vi "战舰弹窗.vi"() -> ()   [LabVIEW 2018]
panel:
  in  "关卡":dbl
  out "失败界面":picture
  out "胜利界面":picture
  out "敌机是否入侵":bool
  out "得分":dbl
  out "战舰爆炸":picture
  out "血量":dbl
  out "战舰血量":T1 scale=0.0..100.0
  out "敌机爆炸":picture
  in  "敌机数量":dbl
  in  "敌机速度":dbl
  out "敌机":picture
  out "按键":dbl
  out "战舰":T2
  out "激光武器1":T3
  out "激光武器 2":T3
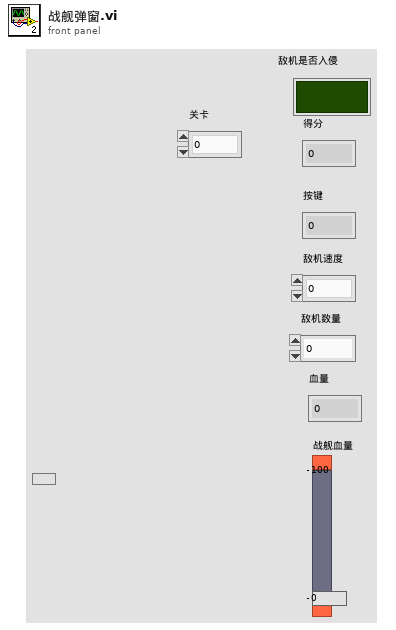
[diagram p1: front panel]
types:
  T1 = typedef "战列巡洋舰_血条.ctl" = dbl
  T2 = typedef "战列巡洋舰.ctl" = picture
  T3 = typedef "战列巡洋舰_激光武器.ctl" = picture
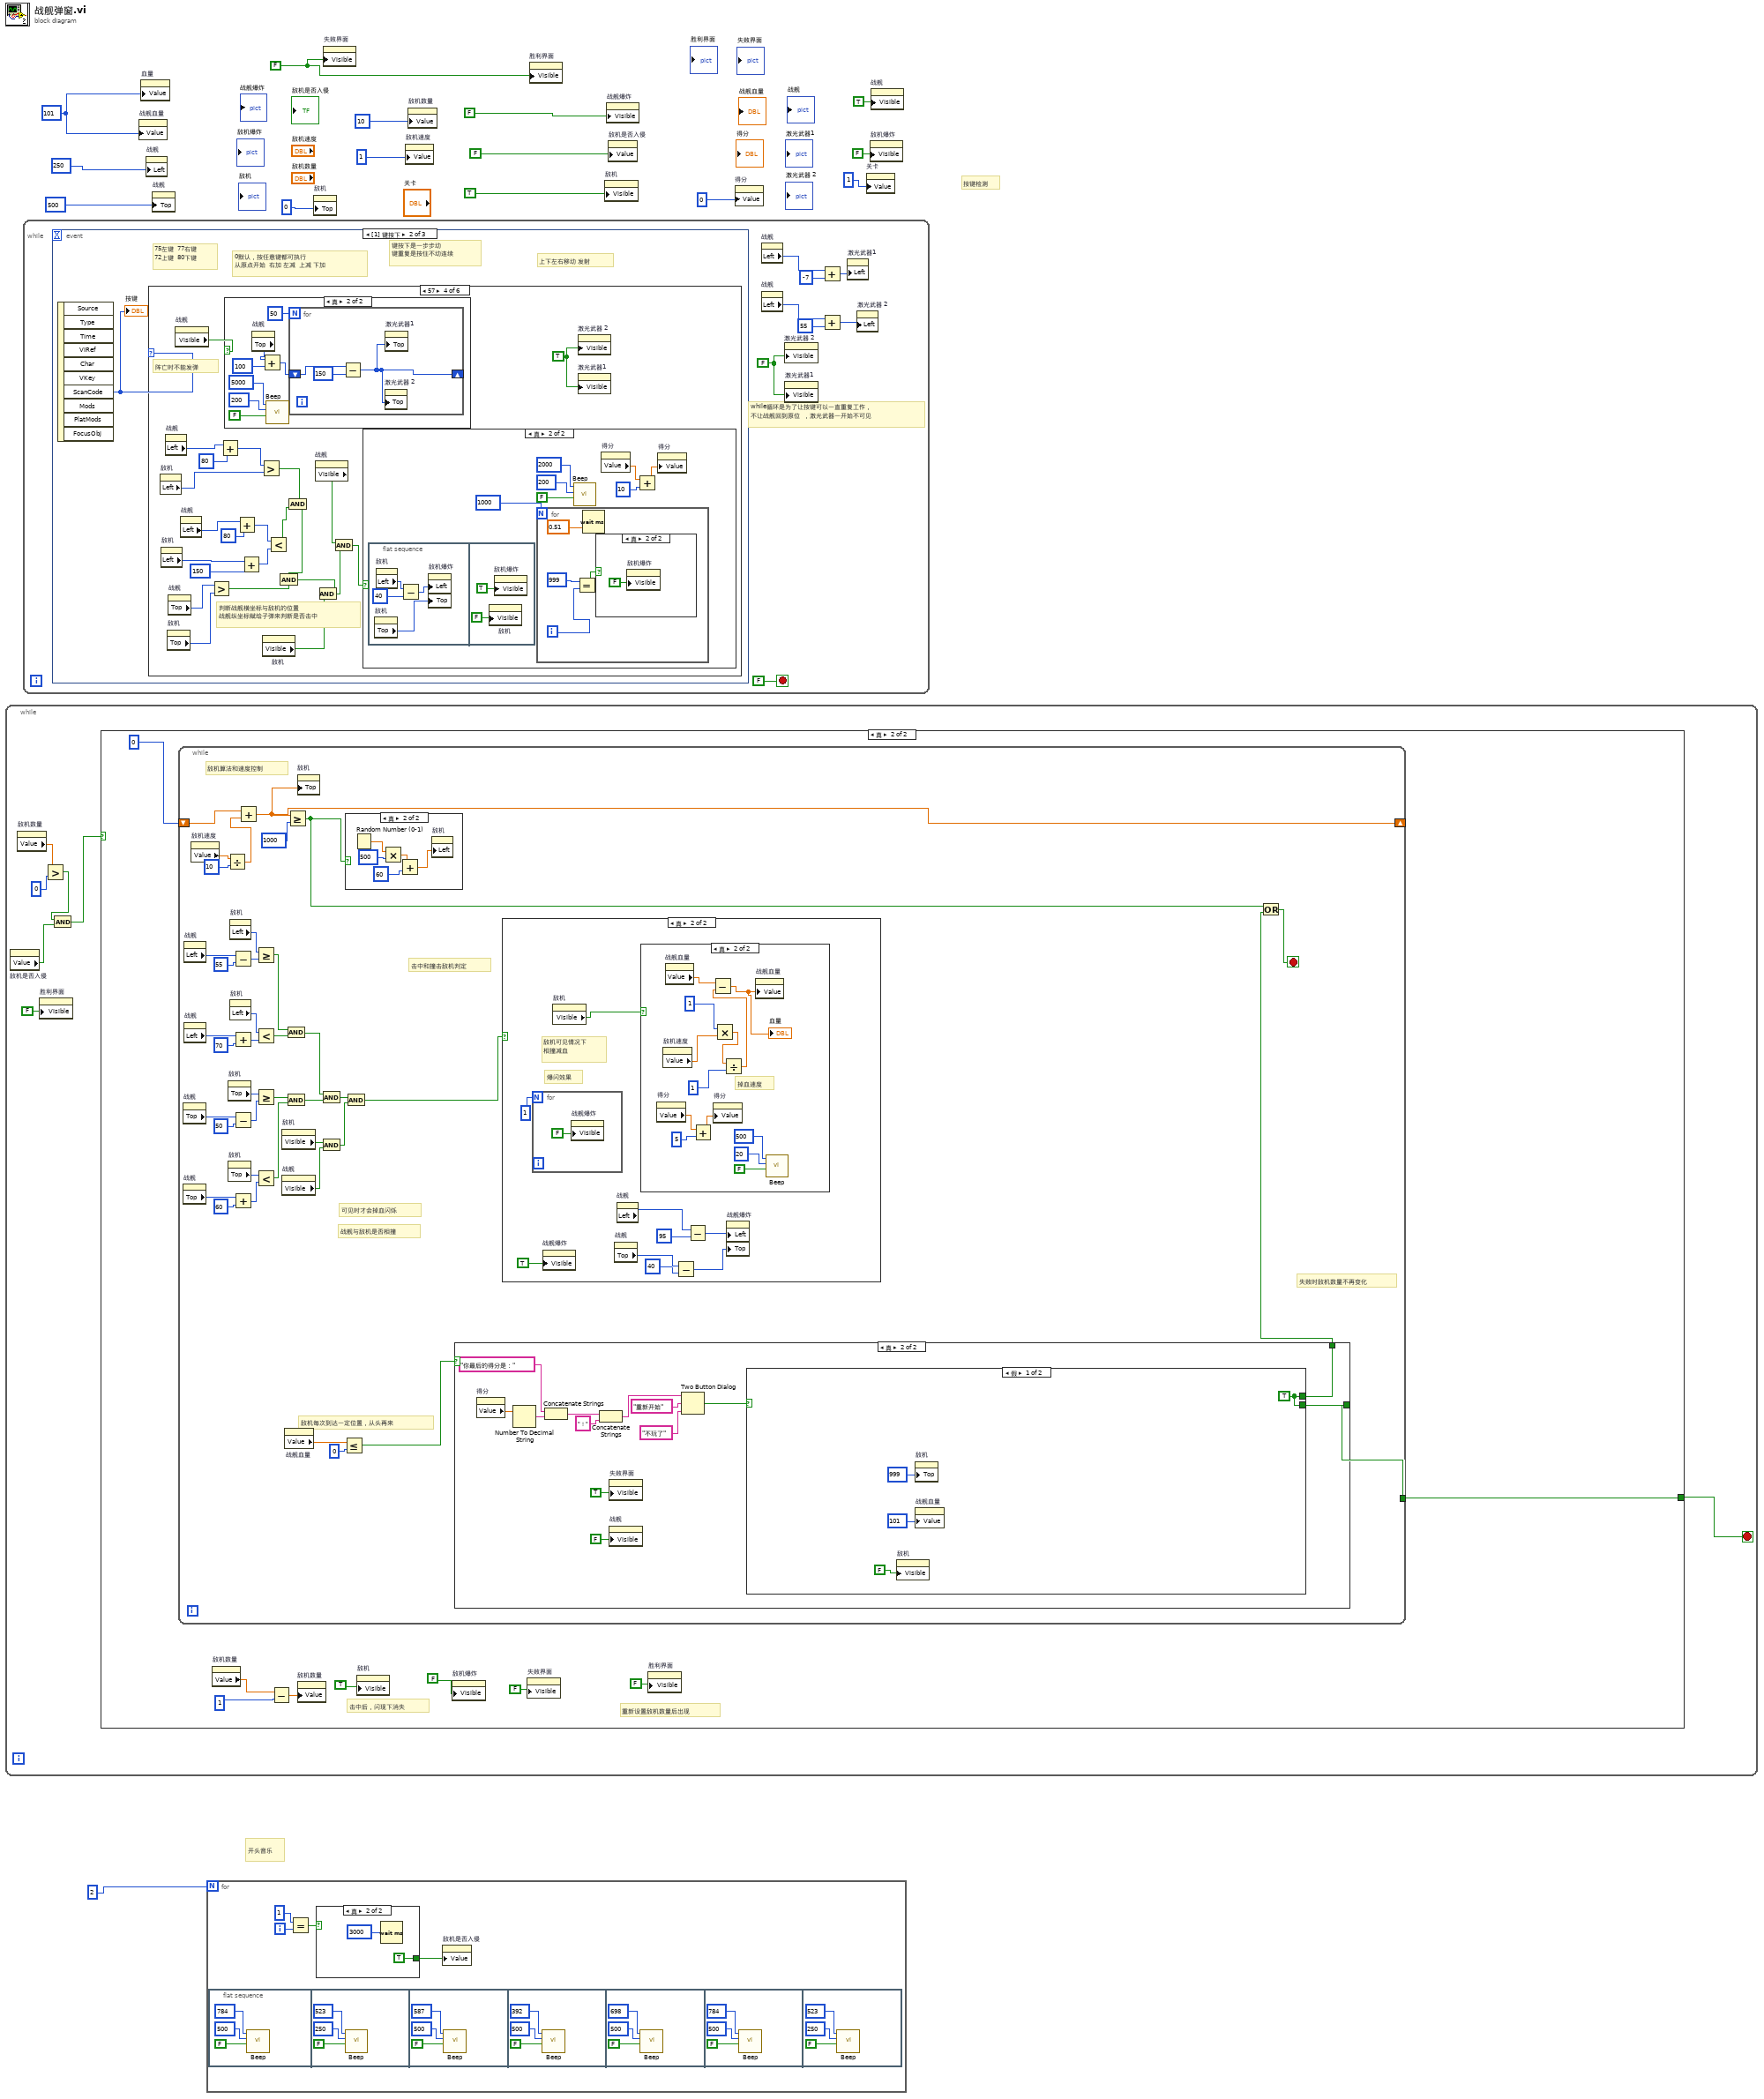
[diagram p0: block diagram]
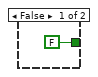
[diagram p2: hidden frame]
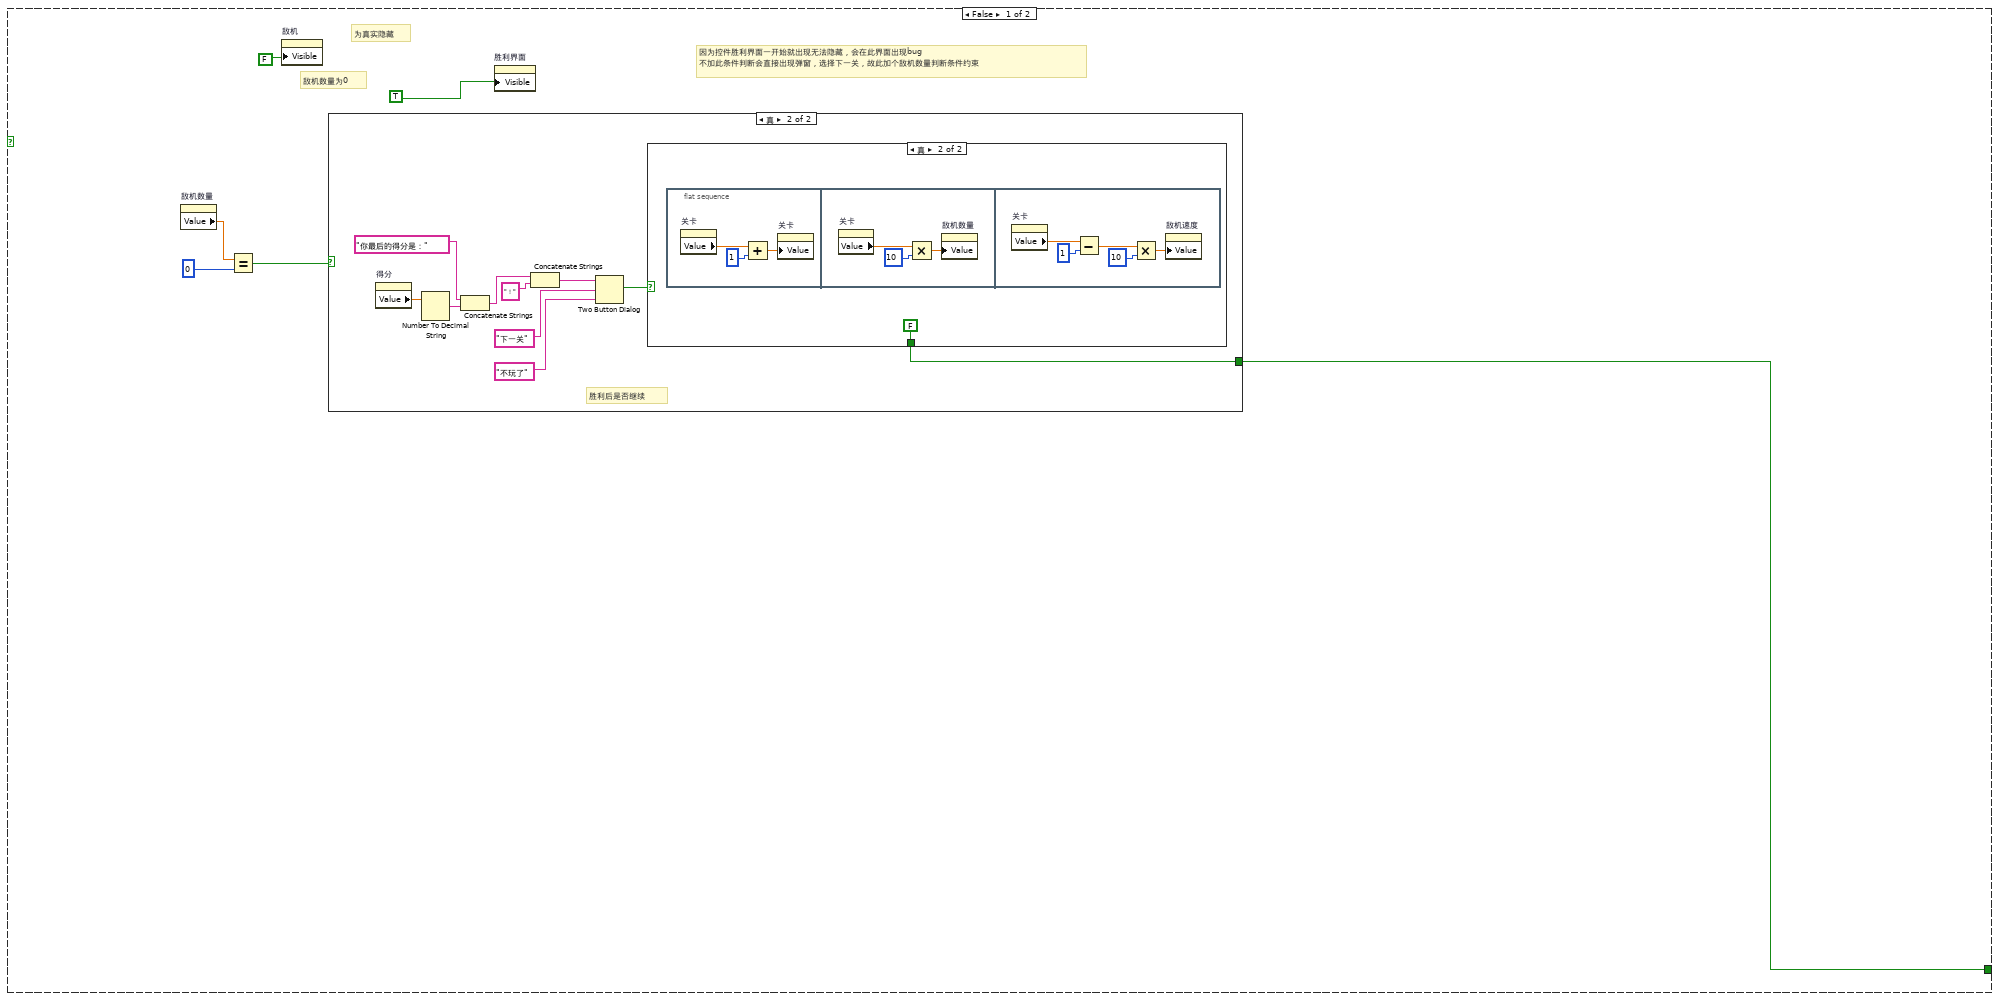
[diagram p3: hidden frame]
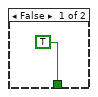
[diagram p5: hidden frame]
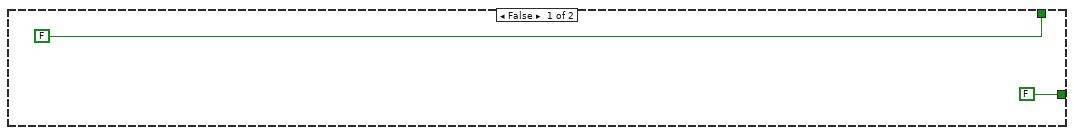
[diagram p6: hidden frame]
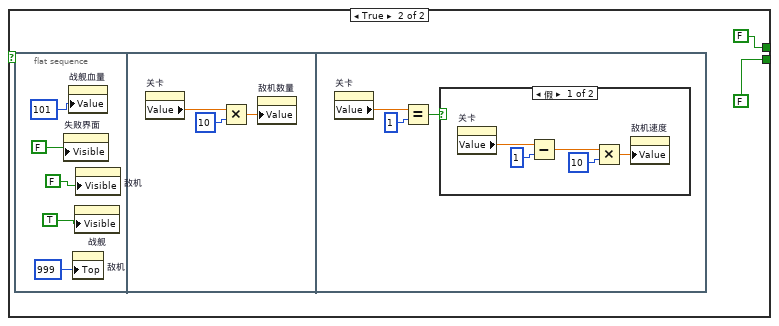
[diagram p7: hidden frame]
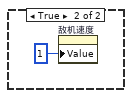
[diagram p8: hidden frame]
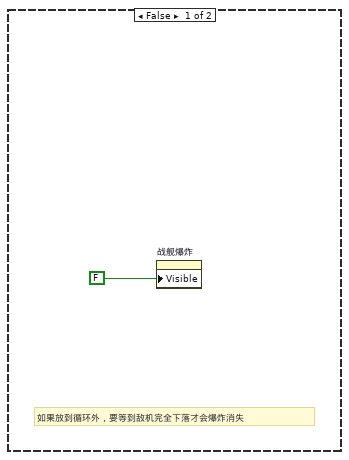
[diagram p9: hidden frame]
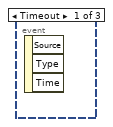
[diagram p12: hidden frame]
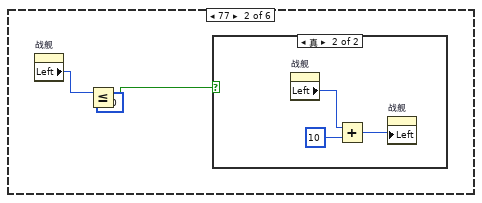
[diagram p14: hidden frame]
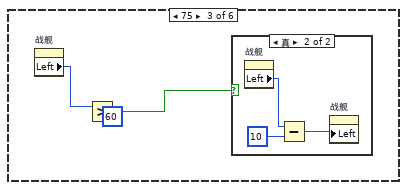
[diagram p16: hidden frame]
diagram:
  w1 = FALSE ("可见")
  w9 = 101
  # "开头音乐"
  # "按键检测"
  n1 = while {
    stop <- w17 stop-if-true
    n2 = property on="敌机是否入侵" class="Bool (严格)"() -> ("Value"=w20:bool)  [unwired: 2 in, 2 out]
    n3 = property on="敌机数量" class="DigNum (严格)"() -> ("Value"=w22:dbl)  [unwired: 2 in, 2 out]
    n4 = property on="胜利界面" class="Pict"("Visible"=FALSE ("可见")) -> ()  [unwired: 2 in, 2 out]
    n5 = Greater?(x=w22, y=0) -> (0:w19:bool)
    n6 = And(x=w19, y=w20) -> (x .and. y?=w18:bool)
    n7 = case shown="真" w18 {
      tunnel: [w26 w53] -> w17
      frame False {
        # "因为控件胜利界面一开始就出现无法隐藏，会在此界面出现bug\n不加此条件判断会直接出现弹窗，选择下一关，故此加个敌机数量判断条件约束"
        # "敌机数量为0"
        # "为真实隐藏"
        n8 = property on="敌机数量" class="DigNum (严格)"() -> ("Value"=w25:dbl)  [unwired: 2 in, 2 out]
        n9 = Equal?(x=w25, y=0) -> (x = y?=w23:bool)
        n10 = property on="敌机" class="Pict"("Visible"=FALSE ("可见")) -> ()  [unwired: 2 in, 2 out]
        n11 = case shown="真" w23 {
          tunnel: [_ w29] -> w26
          frame False {
          }
          frame True {
            # "胜利后是否继续"
            n12 = property on="得分" class="DigNum (严格)"() -> ("Value"=w37:dbl)  [unwired: 2 in, 2 out]
            n13 = Number To Decimal String(number=w37) -> (decimal integer string=w35:string)  [unwired: 1 in]
            n14 = Concatenate Strings("你最后的得分是：", w35) -> (w34:string)
            n15 = Concatenate Strings(w34, "！") -> (w32:string)
            n16 = Two Button Dialog(message=w32, 1:"不玩了" ("F按钮名称（“取消”）"), 2:"下一关" ("T按钮名称（“确定”）")) -> (T button?=w38:bool)
            n17 = case shown="真" w38 {
              tunnel: [TRUE FALSE] -> w29
              frame False {
              }
              frame True {
                n18 = flat-sequence {
                  frame #0 {
                    n19 = property on="关卡" class="DigNum (严格)"() -> ("Value"=w43:dbl)  [unwired: 2 in, 2 out]
                    n20 = Add(x=w43, y=1) -> (x+y=w41:dbl)
                    n21 = property on="关卡" class="DigNum (严格)"("Value"=w41) -> ()  [unwired: 2 in, 2 out]
                  }
                  frame #1 {
                    n22 = property on="关卡" class="DigNum (严格)"() -> ("Value"=w45:dbl)  [unwired: 2 in, 2 out]
                    n23 = Multiply(x=w45, y=10) -> (x*y=w46:dbl)
                    n24 = property on="敌机数量" class="DigNum (严格)"("Value"=w46) -> ()  [unwired: 2 in, 2 out]
                  }
                  frame #2 {
                    n25 = property on="关卡" class="DigNum (严格)"() -> ("Value"=w50:dbl)  [unwired: 2 in, 2 out]
                    n26 = Subtract(x=w50, y=1) -> (x-y=w48:dbl)
                    n27 = Multiply(x=w48, y=10) -> (x*y=w47:dbl)
                    n28 = property on="敌机速度" class="DigNum (严格)"("Value"=w47) -> ()  [unwired: 2 in, 2 out]
                  }
                }
              }
            }
          }
        }
        n29 = property on="胜利界面" class="Pict"("Visible"=TRUE ("可见")) -> ()  [unwired: 2 in, 2 out]
      }
      frame True {
        # "重新设置敌机数量后出现"
        # "击中后，闪现下消失"
        # "敌机每次到达一定位置，从头再来"
        n30 = while {
          shift-right: [w98] -> _
          shift-left: 0 -> [w100]
          tunnel: [w64] -> w53
          stop <- w62 stop-if-true
          # "失败时敌机数量不再变化"
          # "击中和撞击敌机判定"
          # "可见时才会掉血闪烁"
          # "战舰与敌机是否相撞"
          # "敌机算法和速度控制"
          n31 = property on="战舰" class="Pict (严格)"() -> ("Top"=w83:i32)  [unwired: 2 in, 2 out]
          n32 = property on="战舰" class="Pict (严格)"() -> ("Top"=w77:i32)  [unwired: 2 in, 2 out]
          n33 = property on="战舰" class="Pict (严格)"() -> ("Left"=w93:i32)  [unwired: 2 in, 2 out]
          n34 = property on="战舰" class="Pict (严格)"() -> ("Left"=w87:i32)  [unwired: 2 in, 2 out]
          n35 = property on="敌机速度" class="DigNum (严格)"() -> ("Value"=w97:dbl)  [unwired: 2 in, 2 out]
          n36 = Divide(x=w97, y=10) -> (x/y=w96:dbl)
          n37 = property on="敌机" class="Pict"() -> ("Top"=w84:i32)  [unwired: 2 in, 2 out]
          n38 = property on="敌机" class="Pict"() -> ("Top"=w76:i32)  [unwired: 2 in, 2 out]
          n39 = property on="敌机" class="Pict"() -> ("Left"=w94:i32)  [unwired: 2 in, 2 out]
          n40 = property on="敌机" class="Pict"() -> ("Left"=w89:i32)  [unwired: 2 in, 2 out]
          n41 = Subtract(x=w93, y=55) -> (x-y=w92:i32)
          n42 = Add(x=w87, y=70) -> (x+y=w86:i32)
          n43 = Subtract(x=w83, y=50) -> (x-y=w81:i32)
          n44 = Add(x=w77, y=60) -> (x+y=w79:i32)
          n45 = Add(x=w100, y=w96) -> (x+y=w98:dbl)
          n46 = Greater Or Equal?(x=w94, y=w92) -> (x >= y?=w90:bool)
          n47 = Less?(x=w89, y=w86) -> (x < y?=w85:bool)
          n48 = Greater Or Equal?(x=w84, y=w81) -> (x >= y?=w75:bool)
          n49 = Less?(x=w76, y=w79) -> (x < y?=w74:bool)
          n50 = property on="敌机" class="Pict"() -> ("Visible"=w67:bool)  [unwired: 2 in, 2 out]
          n51 = property on="战舰" class="Pict (严格)"() -> ("Visible"=w66:bool)  [unwired: 2 in, 2 out]
          n52 = And(x=w90, y=w85) -> (x .and. y?=w80:bool)
          n53 = And(x=w75, y=w74) -> (x .and. y?=w73:bool)
          n54 = property on="战舰血量" class="Slide (严格)"() -> ("Value"=w69:T1)  [unwired: 2 in, 2 out]
          n55 = Greater Or Equal?(x=w98, y=1000) -> (x >= y?=w63:bool)
          n56 = property on="敌机" class="Pict"("Top"=w98) -> ()  [unwired: 2 in, 2 out]
          n57 = And(x=w80, y=w73) -> (x .and. y?=w72:bool)
          n58 = And(x=w67, y=w66) -> (x .and. y?=w65:bool)
          n59 = Less Or Equal?(x=w69, y=0) -> (x <= y?=w70:bool)
          n60 = case shown="真" w63 {
            frame False {
            }
            frame True {
              n61 = Random Number (0-1)() -> (number: 0 to 1=w167:dbl)
              n62 = Multiply(x=w167, y=500) -> (x*y=w165:dbl)
              n63 = Add(x=w165, y=60) -> (x+y=w164:dbl)
              n64 = property on="敌机" class="Pict"("Left"=w164) -> ()  [unwired: 2 in, 2 out]
            }
          }
          n65 = And(x=w72, y=w65) -> (x .and. y?=w71:bool)
          n66 = case shown="真" w70 {
            tunnel: [FALSE w104] -> w64
            tunnel: [FALSE w103] -> w61
            frame False {
            }
            frame True {
              n67 = property on="得分" class="DigNum (严格)"() -> ("Value"=w115:dbl)  [unwired: 2 in, 2 out]
              n68 = Number To Decimal String(number=w115) -> (decimal integer string=w114:string)  [unwired: 1 in]
              n69 = Concatenate Strings("你最后的得分是：", w114) -> (w113:string)
              n70 = Concatenate Strings(w113, "！") -> (w112:string)
              n71 = property on="失败界面" class="Pict"("Visible"=TRUE ("可见")) -> ()  [unwired: 2 in, 2 out]
              n72 = property on="战舰" class="Pict (严格)"("Visible"=FALSE ("可见")) -> ()  [unwired: 2 in, 2 out]
              n73 = Two Button Dialog(message=w112, 1:"不玩了" ("F按钮名称（“取消”）"), 2:"重新开始" ("T按钮名称（“确定”）")) -> (T button?=w107:bool)
              n74 = case shown="假" w107 {
                tunnel: [w117 FALSE] -> w104
                tunnel: [w117 FALSE] -> w103
                frame False {
                  w117 = TRUE
                  n75 = property on="敌机" class="Pict"("Visible"=FALSE ("可见")) -> ()  [unwired: 2 in, 2 out]
                  n76 = property on="敌机" class="Pict"("Top"=999 ("位置:置顶")) -> ()  [unwired: 2 in, 2 out]
                  n77 = property on="战舰血量" class="Slide (严格)"("Value"=101) -> ()  [unwired: 2 in, 2 out]
                }
                frame True {
                  n78 = flat-sequence {
                    frame #0 {
                      n79 = property on="失败界面" class="Pict"("Visible"=FALSE ("可见")) -> ()  [unwired: 2 in, 2 out]
                      n80 = property on="战舰血量" class="Slide (严格)"("Value"=101) -> ()  [unwired: 2 in, 2 out]
                      n81 = property on="敌机" class="Pict"("Top"=999 ("位置:置顶")) -> ()  [unwired: 2 in, 2 out]
                      n82 = property on="战舰" class="Pict (严格)"("Visible"=TRUE ("可见")) -> ()  [unwired: 2 in, 2 out]
                      n83 = property on="敌机" class="Pict"("Visible"=FALSE ("可见")) -> ()  [unwired: 2 in, 2 out]
                    }
                    frame #1 {
                      n84 = property on="关卡" class="DigNum (严格)"() -> ("Value"=w127:dbl)  [unwired: 2 in, 2 out]
                      n85 = Multiply(x=w127, y=10) -> (x*y=w129:dbl)
                      n86 = property on="敌机数量" class="DigNum (严格)"("Value"=w129) -> ()  [unwired: 2 in, 2 out]
                    }
                    frame #2 {
                      n87 = property on="关卡" class="DigNum (严格)"() -> ("Value"=w132:dbl)  [unwired: 2 in, 2 out]
                      n88 = Equal?(x=w132, y=1) -> (x = y?=w130:bool)
                      n89 = case shown="假" w130 {
                        frame False {
                          n90 = property on="关卡" class="DigNum (严格)"() -> ("Value"=w136:dbl)  [unwired: 2 in, 2 out]
                          n91 = Subtract(x=w136, y=1) -> (x-y=w133:dbl)
                          n92 = Multiply(x=w133, y=10) -> (x*y=w137:dbl)
                          n93 = property on="敌机速度" class="DigNum (严格)"("Value"=w137) -> ()  [unwired: 2 in, 2 out]
                        }
                        frame True {
                          n94 = property on="敌机速度" class="DigNum (严格)"("Value"=1) -> ()  [unwired: 2 in, 2 out]
                        }
                      }
                    }
                  }
                }
              }
            }
          }
          n95 = case shown="真" w71 {
            frame False {
              # "如果放到循环外，要等到敌机完全下落才会爆炸消失"
              n96 = property on="战舰爆炸" class="Pict"("Visible"=FALSE ("可见")) -> ()  [unwired: 2 in, 2 out]
            }
            frame True {
              # "爆闪效果"
              # "敌机可见情况下\n相撞减血"
              n97 = for {
                N: 1 -> [_]
                n98 = property on="战舰爆炸" class="Pict"("Visible"=FALSE ("可见")) -> ()  [unwired: 2 in, 2 out]
              }
              n99 = property on="战舰爆炸" class="Pict"("Visible"=TRUE ("可见")) -> ()  [unwired: 2 in, 2 out]
              n100 = property on="敌机" class="Pict"() -> ("Visible"=w148:bool)  [unwired: 2 in, 2 out]
              n101 = property on="战舰" class="Pict (严格)"() -> ("Top"=w143:i32)  [unwired: 2 in, 2 out]
              n102 = property on="战舰" class="Pict (严格)"() -> ("Left"=w146:i32)  [unwired: 2 in, 2 out]
              n103 = case shown="真" w148 {
                frame False {
                }
                frame True {
                  # "掉血速度"
                  n104 = property on="得分" class="DigNum (严格)"() -> ("Value"=w155:dbl)  [unwired: 2 in, 2 out]
                  n105 = property on="敌机速度" class="DigNum (严格)"() -> ("Value"=w161:dbl)  [unwired: 2 in, 2 out]
                  n106 = property on="战舰血量" class="Slide (严格)"() -> ("Value"=w162:T1)  [unwired: 2 in, 2 out]
                  n107 = Add(x=w155, y=5) -> (x+y=w154:dbl)
                  n108 = Multiply(x=1, y=w161) -> (x*y=w160:dbl)
                  n109 = property on="得分" class="DigNum (严格)"("Value"=w154) -> ()  [unwired: 2 in, 2 out]
                  n110 = Divide(x=w160, y=1) -> (x/y=w157:dbl)
                  n111 = Subtract(x=w162, y=w157) -> (x-y=w156:T1)
                  "血量" <- w156
                  n112 = property on="战舰血量" class="Slide (严格)"("Value"=w156) -> ()  [unwired: 2 in, 2 out]
                  n113 = call <vilib>:"Beep.vi"("use system alert? (T)"=FALSE, "duration (msec)"=u32 20, "frequency (Hz)"=u32 500) -> ()  [unwired: 9 in]
                }
              }
              n114 = Subtract(x=w143, y=40) -> (x-y=w141:i32)
              n115 = Subtract(x=w146, y=95) -> (x-y=w144:i32)
              n116 = property on="战舰爆炸" class="Pict"("Left"=w144, "Top"=w141) -> ()  [unwired: 2 in, 2 out]
            }
          }
          n117 = Or(x=w63, y=w61) -> (x .or. y?=w62:bool)
        }
        n118 = property on="敌机数量" class="DigNum (严格)"() -> ("Value"=w58:dbl)  [unwired: 2 in, 2 out]
        n119 = Subtract(x=w58, y=1) -> (x-y=w59:dbl)
        n120 = property on="敌机数量" class="DigNum (严格)"("Value"=w59) -> ()  [unwired: 2 in, 2 out]
        n121 = property on="敌机" class="Pict"("Visible"=TRUE ("可见")) -> ()  [unwired: 2 in, 2 out]
        n122 = property on="敌机爆炸" class="Pict"("Visible"=FALSE ("可见")) -> ()  [unwired: 2 in, 2 out]
        n123 = property on="失败界面" class="Pict"("Visible"=FALSE ("可见")) -> ()  [unwired: 2 in, 2 out]
        n124 = property on="胜利界面" class="Pict"("Visible"=FALSE ("可见")) -> ()  [unwired: 2 in, 2 out]
      }
    }
  }
  n125 = while {
    stop <- FALSE stop-if-true
    w168 = FALSE
    # "while循环是为了让按键可以一直重复工作，\n不让战舰回到原位  ，激光武器一开始不可见"
    n126 = event shown="[1] 键按下" {
      selector: _ -> [_ _ _]
      dyn-events: _ -> [_ _ _]
      timeout: _ -> [_ _ _]
      event Timeout {
        n127 = event-data() -> ()  [unwired: 1 in, 3 out]
      }
      event Key Down {
        # "上下左右移动 发射"
        # "键按下是一步步动\n键重复是按住不动连续"
        # "75左键  77右键\n72上键  80下键"
        # "0默认，按任意键都可执行\n从原点开始  右加 左减  上减 下加"
        n128 = event-data() -> ("ScanCode"=w176:i16)  [unwired: 1 in, 9 out]
        "按键" <- w176
        n129 = case shown="57" w176 {
          frame 0, Default {
          }
          frame 77 {
            n130 = property on="战舰" class="Pict (严格)"() -> ("Left"=w179:i32)  [unwired: 2 in, 2 out]
            n131 = Less Or Equal?(x=w179, y=500) -> (x <= y?=w177:bool)
            n132 = case shown="真" w177 {
              frame False {
              }
              frame True {
                n133 = property on="战舰" class="Pict (严格)"() -> ("Left"=w181:i32)  [unwired: 2 in, 2 out]
                n134 = Add(x=w181, y=10) -> (x+y=w182:i32)
                n135 = property on="战舰" class="Pict (严格)"("Left"=w182) -> ()  [unwired: 2 in, 2 out]
              }
            }
          }
          frame 75 {
            n136 = property on="战舰" class="Pict (严格)"() -> ("Left"=w185:i32)  [unwired: 2 in, 2 out]
            n137 = Greater?(x=w185, y=60) -> (0:w183:bool)
            n138 = case shown="真" w183 {
              frame False {
              }
              frame True {
                n139 = property on="战舰" class="Pict (严格)"() -> ("Left"=w187:i32)  [unwired: 2 in, 2 out]
                n140 = Subtract(x=w187, y=10) -> (x-y=w188:i32)
                n141 = property on="战舰" class="Pict (严格)"("Left"=w188) -> ()  [unwired: 2 in, 2 out]
              }
            }
          }
          frame 57 {
            w211 = TRUE
            # "阵亡时不能发弹"
            # "判断战舰横坐标与敌机的位置\n战舰纵坐标赋给子弹来判断是否击中"
            n142 = property on="敌机" class="Pict"() -> ("Left"=w208:i32)  [unwired: 2 in, 2 out]
            n143 = property on="敌机" class="Pict"() -> ("Left"=w201:i32)  [unwired: 2 in, 2 out]
            n144 = property on="战舰" class="Pict (严格)"() -> ("Left"=w210:i32)  [unwired: 2 in, 2 out]
            n145 = property on="敌机" class="Pict"() -> ("Top"=w195:i32)  [unwired: 2 in, 2 out]
            n146 = property on="战舰" class="Pict (严格)"() -> ("Top"=w196:i32)  [unwired: 2 in, 2 out]
            n147 = property on="战舰" class="Pict (严格)"() -> ("Visible"=w189:bool)  [unwired: 2 in, 2 out]
            n148 = property on="战舰" class="Pict (严格)"() -> ("Left"=w203:i32)  [unwired: 2 in, 2 out]
            n149 = Greater?(x=w196, y=w195) -> (0:w197:bool)
            n150 = Add(x=w210, y=80) -> (x+y=w207:i32)
            n151 = case shown="真" w189 {
              frame False {
              }
              frame True {
                n152 = property on="战舰" class="Pict (严格)"() -> ("Top"=w217:i32)  [unwired: 2 in, 2 out]
                n153 = Add(x=w217, y=100) -> (x+y=w215:i32)
                n154 = call <vilib>:"Beep.vi"("use system alert? (T)"=FALSE, "duration (msec)"=u32 200, "frequency (Hz)"=u32 5000) -> ()  [unwired: 9 in]
                n155 = for {
                  N: 50 -> [_]
                  shift-right: [w219] -> _
                  shift-left: w215 -> [w221]
                  n156 = Subtract(x=w221, y=150) -> (x-y=w219:i32)
                  n157 = property on="激光武器 2" class="Pict (严格)"("Top"=w219) -> ()  [unwired: 2 in, 2 out]
                  n158 = property on="激光武器1" class="Pict (严格)"("Top"=w219) -> ()  [unwired: 2 in, 2 out]
                }
              }
            }
            n159 = Add(x=w203, y=80) -> (x+y=w205:i32)
            n160 = Add(x=w201, y=150) -> (x+y=w200:i32)
            n161 = Greater?(x=w207, y=w208) -> (0:w206:bool)
            n162 = property on="敌机" class="Pict"() -> ("Visible"=w193:bool)  [unwired: 2 in, 2 out]
            n163 = Less?(x=w205, y=w200) -> (x < y?=w202:bool)
            n164 = And(x=w206, y=w202) -> (x .and. y?=w198:bool)
            n165 = And(x=w198, y=w197) -> (x .and. y?=w194:bool)
            n166 = property on="战舰" class="Pict (严格)"() -> ("Visible"=w192:bool)  [unwired: 2 in, 2 out]
            n167 = And(x=w194, y=w193) -> (x .and. y?=w191:bool)
            n168 = And(x=w192, y=w191) -> (x .and. y?=w190:bool)
            n169 = case shown="真" w190 {
              frame False {
              }
              frame True {
                n170 = flat-sequence {
                  frame #0 {
                    n171 = property on="敌机" class="Pict"() -> ("Top"=w232:i32)  [unwired: 2 in, 2 out]
                    n172 = property on="敌机" class="Pict"() -> ("Left"=w230:i32)  [unwired: 2 in, 2 out]
                    n173 = Subtract(x=w230, y=40) -> (x-y=w229:i32)
                    n174 = property on="敌机爆炸" class="Pict"("Left"=w229, "Top"=w232) -> ()  [unwired: 2 in, 2 out]
                  }
                  frame #1 {
                    n175 = property on="敌机" class="Pict"("Visible"=FALSE ("可见")) -> ()  [unwired: 2 in, 2 out]
                    n176 = property on="敌机爆炸" class="Pict"("Visible"=TRUE ("可见")) -> ()  [unwired: 2 in, 2 out]
                  }
                }
                n177 = for {
                  N: 1000 -> [_]
                  i -> [w237]
                  n178 = Equal?(x=999, y=w237) -> (x = y?=w238:bool)
                  n179 = Wait (ms)(milliseconds to wait=0.51) -> ()  [unwired: 1 out]
                  n180 = case shown="真" w238 {
                    frame False {
                    }
                    frame True {
                      n181 = property on="敌机爆炸" class="Pict"("Visible"=FALSE ("可见")) -> ()  [unwired: 2 in, 2 out]
                    }
                  }
                }
                n182 = call <vilib>:"Beep.vi"("use system alert? (T)"=FALSE, "duration (msec)"=u32 200, "frequency (Hz)"=u32 2000) -> ()  [unwired: 9 in]
                n183 = property on="得分" class="DigNum (严格)"() -> ("Value"=w227:dbl)  [unwired: 2 in, 2 out]
                n184 = Add(x=w227, y=10) -> (x+y=w225:dbl)
                n185 = property on="得分" class="DigNum (严格)"("Value"=w225) -> ()  [unwired: 2 in, 2 out]
              }
            }
            n186 = property on="激光武器 2" class="Pict (严格)"("Visible"=w211) -> ()  [unwired: 2 in, 2 out]
            n187 = property on="激光武器1" class="Pict (严格)"("Visible"=w211) -> ()  [unwired: 2 in, 2 out]
          }
          frame 80 {
            n188 = property on="战舰" class="Pict (严格)"() -> ("Top"=w242:i32)  [unwired: 2 in, 2 out]
            n189 = Less?(x=w242, y=525) -> (x < y?=w240:bool)
            n190 = case shown="真" w240 {
              frame False {
              }
              frame True {
                n191 = property on="战舰" class="Pict (严格)"() -> ("Top"=w244:i32)  [unwired: 2 in, 2 out]
                n192 = Add(x=w244, y=10) -> (x+y=w243:i32)
                n193 = property on="战舰" class="Pict (严格)"("Top"=w243) -> ()  [unwired: 2 in, 2 out]
              }
            }
          }
          frame 72 {
            n194 = property on="战舰" class="Pict (严格)"() -> ("Top"=w248:i32)  [unwired: 2 in, 2 out]
            n195 = Greater Or Equal?(x=w248, y=25) -> (x >= y?=w247:bool)
            n196 = case shown="真" w247 {
              frame False {
              }
              frame True {
                n197 = property on="战舰" class="Pict (严格)"() -> ("Top"=w251:i32)  [unwired: 2 in, 2 out]
                n198 = Subtract(x=w251, y=10) -> (x-y=w250:i32)
                n199 = property on="战舰" class="Pict (严格)"("Top"=w250) -> ()  [unwired: 2 in, 2 out]
              }
            }
          }
        }
      }
      event Key Repeat {
        # "75左键  77右键\n72上键  80下键\n空格 57"
        # "0默认，按任意键都可执行\n从原点开始  右加 左减  上减 下加"
        n200 = event-data() -> ("ScanCode"=w252:i16)  [unwired: 1 in, 9 out]
        n201 = case shown="72" w252 {
          frame 0, Default {
          }
          frame 77 {
            n202 = property on="战舰" class="Pict (严格)"() -> ("Left"=w255:i32)  [unwired: 2 in, 2 out]
            n203 = Less Or Equal?(x=w255, y=500) -> (x <= y?=w254:bool)
            n204 = case shown="真" w254 {
              frame False {
              }
              frame True {
                n205 = property on="战舰" class="Pict (严格)"() -> ("Left"=w257:i32)  [unwired: 2 in, 2 out]
                n206 = Add(x=w257, y=10) -> (x+y=w258:i32)
                n207 = property on="战舰" class="Pict (严格)"("Left"=w258) -> ()  [unwired: 2 in, 2 out]
              }
            }
          }
          frame 75 {
            n208 = property on="战舰" class="Pict (严格)"() -> ("Left"=w261:i32)  [unwired: 2 in, 2 out]
            n209 = Greater Or Equal?(x=w261, y=25) -> (x >= y?=w260:bool)
            n210 = case shown="真" w260 {
              frame False {
              }
              frame True {
                n211 = property on="战舰" class="Pict (严格)"() -> ("Left"=w264:i32)  [unwired: 2 in, 2 out]
                n212 = Subtract(x=w264, y=10) -> (x-y=w263:i32)
                n213 = property on="战舰" class="Pict (严格)"("Left"=w263) -> ()  [unwired: 2 in, 2 out]
              }
            }
          }
          frame 80 {
            n214 = property on="战舰" class="Pict (严格)"() -> ("Top"=w267:i32)  [unwired: 2 in, 2 out]
            n215 = Less Or Equal?(x=w267, y=525) -> (x <= y?=w266:bool)
            n216 = case shown="真" w266 {
              frame False {
              }
              frame True {
                n217 = property on="战舰" class="Pict (严格)"() -> ("Top"=w269:i32)  [unwired: 2 in, 2 out]
                n218 = Add(x=w269, y=10) -> (x+y=w268:i32)
                n219 = property on="战舰" class="Pict (严格)"("Top"=w268) -> ()  [unwired: 2 in, 2 out]
              }
            }
          }
          frame 72 {
            n220 = property on="战舰" class="Pict (严格)"() -> ("Top"=w273:i32)  [unwired: 2 in, 2 out]
            n221 = Greater Or Equal?(x=w273, y=25) -> (x >= y?=w272:bool)
            n222 = case shown="真" w272 {
              frame False {
              }
              frame True {
                n223 = property on="战舰" class="Pict (严格)"() -> ("Top"=w276:i32)  [unwired: 2 in, 2 out]
                n224 = Subtract(x=w276, y=10) -> (x-y=w275:i32)
                n225 = property on="战舰" class="Pict (严格)"("Top"=w275) -> ()  [unwired: 2 in, 2 out]
              }
            }
          }
        }
      }
    }
    n226 = property on="战舰" class="Pict (严格)"() -> ("Left"=w174:i32)  [unwired: 2 in, 2 out]
    n227 = property on="战舰" class="Pict (严格)"() -> ("Left"=w170:i32)  [unwired: 2 in, 2 out]
    n228 = property on="激光武器 2" class="Pict (严格)"("Visible"=w168) -> ()  [unwired: 2 in, 2 out]
    n229 = property on="激光武器1" class="Pict (严格)"("Visible"=w168) -> ()  [unwired: 2 in, 2 out]
    n230 = Add(x=w174, y=-7) -> (x+y=w173:i32)
    n231 = Add(x=w170, y=55) -> (x+y=w169:i32)
    n232 = property on="激光武器1" class="Pict (严格)"("Left"=w173) -> ()  [unwired: 2 in, 2 out]
    n233 = property on="激光武器 2" class="Pict (严格)"("Left"=w169) -> ()  [unwired: 2 in, 2 out]
  }
  n234 = property on="战舰血量" class="Slide (严格)"("Value"=w9) -> ()  [unwired: 2 in, 2 out]
  n235 = property on="血量" class="DigNum (严格)"("Value"=w9) -> ()  [unwired: 2 in, 2 out]
  n236 = property on="战舰" class="Pict (严格)"("Left"=250 ("位置:居左")) -> ()  [unwired: 2 in, 2 out]
  n237 = property on="战舰" class="Pict (严格)"("Top"=500 ("位置:置顶")) -> ()  [unwired: 2 in, 2 out]
  n238 = for {
    N: 2 -> [_]
    i -> [w278]
    n239 = flat-sequence {
      frame #0 {
        n240 = call <vilib>:"Beep.vi"("use system alert? (T)"=FALSE, "duration (msec)"=500, "frequency (Hz)"=784) -> ()  [unwired: 9 in]
      }
      frame #1 {
        n241 = call <vilib>:"Beep.vi"("use system alert? (T)"=FALSE, "duration (msec)"=250, "frequency (Hz)"=523) -> ()  [unwired: 9 in]
      }
      frame #2 {
        n242 = call <vilib>:"Beep.vi"("use system alert? (T)"=FALSE, "duration (msec)"=500, "frequency (Hz)"=587) -> ()  [unwired: 9 in]
      }
      frame #3 {
        n243 = call <vilib>:"Beep.vi"("use system alert? (T)"=FALSE, "duration (msec)"=500, "frequency (Hz)"=392) -> ()  [unwired: 9 in]
      }
      frame #4 {
        n244 = call <vilib>:"Beep.vi"("use system alert? (T)"=FALSE, "duration (msec)"=500, "frequency (Hz)"=698) -> ()  [unwired: 9 in]
      }
      frame #5 {
        n245 = call <vilib>:"Beep.vi"("use system alert? (T)"=FALSE, "duration (msec)"=500, "frequency (Hz)"=784) -> ()  [unwired: 9 in]
      }
      frame #6 {
        n246 = call <vilib>:"Beep.vi"("use system alert? (T)"=FALSE, "duration (msec)"=250, "frequency (Hz)"=523) -> ()  [unwired: 9 in]
      }
    }
    n247 = Equal?(x=1, y=w278) -> (x = y?=w280:bool)
    n248 = case shown="真" w280 {
      tunnel: [FALSE ("敌机是否入侵") TRUE ("敌机是否入侵")] -> w277
      frame False {
      }
      frame True {
        n249 = Wait (ms)(milliseconds to wait=u32 3000 ("等待时间（毫秒）")) -> ()  [unwired: 1 out]
      }
    }
    n250 = property on="敌机是否入侵" class="Bool (严格)"("Value"=w277) -> ()  [unwired: 2 in, 2 out]
  }
  n251 = property on="敌机" class="Pict"("Top"=0) -> ()  [unwired: 2 in, 2 out]
  n252 = property on="失败界面" class="Pict"("Visible"=w1) -> ()  [unwired: 2 in, 2 out]
  n253 = property on="敌机速度" class="DigNum (严格)"("Value"=1) -> ()  [unwired: 2 in, 2 out]
  n254 = property on="敌机数量" class="DigNum (严格)"("Value"=10) -> ()  [unwired: 2 in, 2 out]
  n255 = property on="胜利界面" class="Pict"("Visible"=w1) -> ()  [unwired: 2 in, 2 out]
  n256 = property on="敌机" class="Pict"("Visible"=TRUE ("可见")) -> ()  [unwired: 2 in, 2 out]
  n257 = property on="战舰爆炸" class="Pict"("Visible"=FALSE ("可见")) -> ()  [unwired: 2 in, 2 out]
  n258 = property on="敌机是否入侵" class="Bool (严格)"("Value"=FALSE ("敌机是否入侵")) -> ()  [unwired: 2 in, 2 out]
  n259 = property on="得分" class="DigNum (严格)"("Value"=0) -> ()  [unwired: 2 in, 2 out]
  n260 = property on="关卡" class="DigNum (严格)"("Value"=1) -> ()  [unwired: 2 in, 2 out]
  n261 = property on="敌机爆炸" class="Pict"("Visible"=FALSE ("可见")) -> ()  [unwired: 2 in, 2 out]
  n262 = property on="战舰" class="Pict (严格)"("Visible"=TRUE ("可见")) -> ()  [unwired: 2 in, 2 out]
